vi "stroke_rate.vi"(9 "dt":dbl, 11 "minus-plus":bool[](array[boolean])) -> (3 "stroke rate":dbl[](array[numeric]))   [LabVIEW 2020]
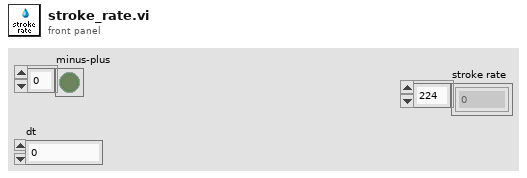
[diagram p1: front panel]
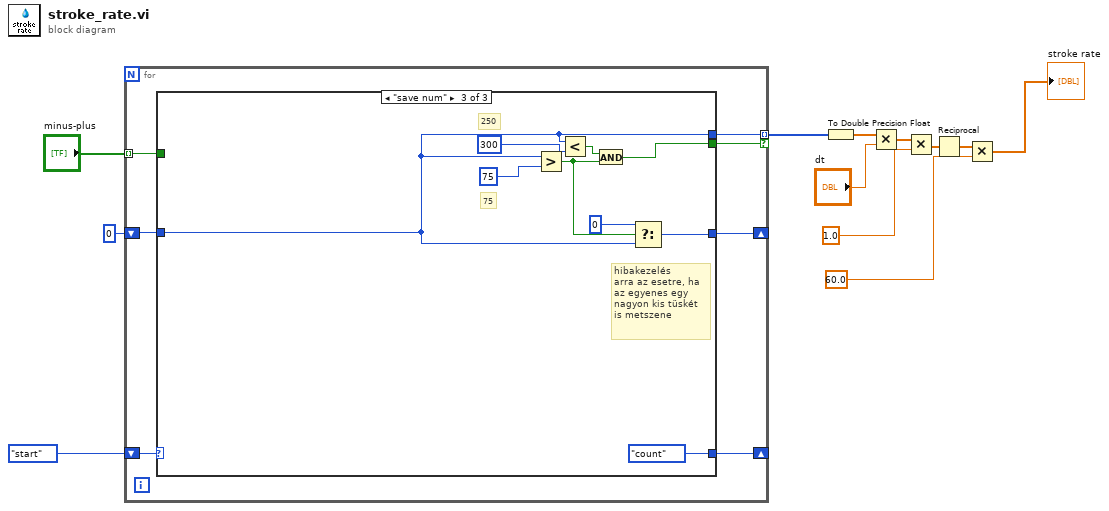
[diagram p0: block diagram]
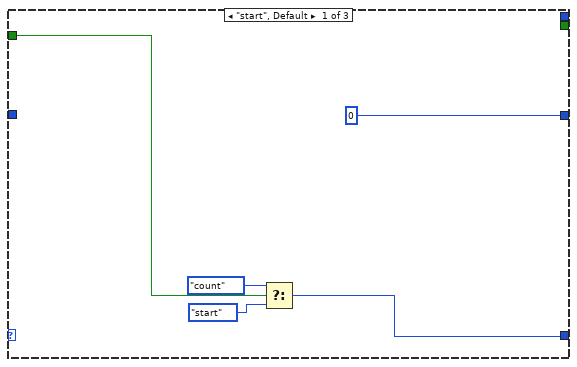
[diagram p2: hidden frame]
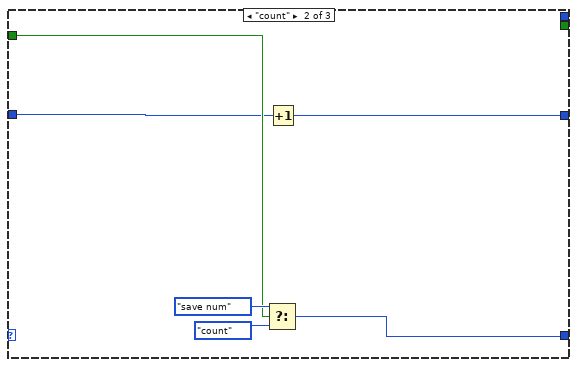
[diagram p3: hidden frame]
diagram:
  n1 = for {
    tunnel: "minus-plus" -> [w18] mode=indexing
    shift-right: [w17] -> _
    shift-left: enum16{"start", "count", "save num"}."start" -> [w19]
    shift-right: [w16] -> _
    shift-left: 0 -> [w15]
    tunnel: [w14] -> w10 mode=indexing if=w13
    n2 = case shown="\"save num\"" w19 {
      tunnel: w18 -> [w24 w29 _]
      tunnel: [w21 w28 enum16{"start", "count", "save num"}."count" ("f")] -> w17
      tunnel: [0 w25 w36] -> w16
      tunnel: w15 -> [_ w26 w32]
      tunnel: [_ _ w32] -> w14
      tunnel: [_ _ w31] -> w13
      frame "start", Default {
        n3 = Select(t=enum16{"start", "count", "save num"}."count", s=w24, f=enum16{"start", "count", "save num"}."start") -> (s? t:f=w21:enum16{"start", "count", "save num"})
      }
      frame "count" {
        n4 = Select(t=enum16{"start", "count", "save num"}."save num", s=w29, f=enum16{"start", "count", "save num"}."count") -> (s? t:f=w28:enum16{"start", "count", "save num"})
        n5 = Increment(x=w26) -> (x+1=w25:i32)
      }
      frame "save num" {
        # "250"
        # "75"
        # "hibakezelés\narra az esetre, ha\naz egyenes egy\nnagyon kis tüskét \nis metszene"
        n6 = Greater?(x=w32, y=75) -> (0:w35:bool)
        n7 = Less?(x=w32, y=300) -> (x < y?=w34:bool)
        n8 = And(x=w34, y=w35) -> (x .and. y?=w31:bool)
        n9 = Select(t=0, s=w35, f=w32) -> (s? t:f=w36:i32)
      }
    }
  }
  n10 = To Double Precision Float(number=w10) -> (double precision float=w9:dbl[])
  n11 = Multiply(x=w9, y="dt") -> (x*y=w8:dbl[])
  n12 = Multiply(x=w8, y=1.0) -> (x*y=w2:dbl[])
  n13 = Reciprocal(x=w2) -> (1/x=w3:dbl[])
  n14 = Multiply(x=w3, y=60.0) -> (x*y=→"stroke rate":dbl[])
